vi "Acquire.Intermediary.vi"(7 "type":T1, 8 "error in":errorcluster, 10 "index":u64, 11 "camera.nit in":refnum<class "camera.lvclass">) -> (0 "error out":errorcluster, 2 "buffer":u16[][](array[numeric]))   [LabVIEW 2020, in "camera.lvclass"]
uses:
  camera.lvclass
  _controls/imageType.ctl
  camera.lvclass/camera.ctl
  lib/O-PL.dll
panel:
  out "Intensity Graph":u16[][](graph)
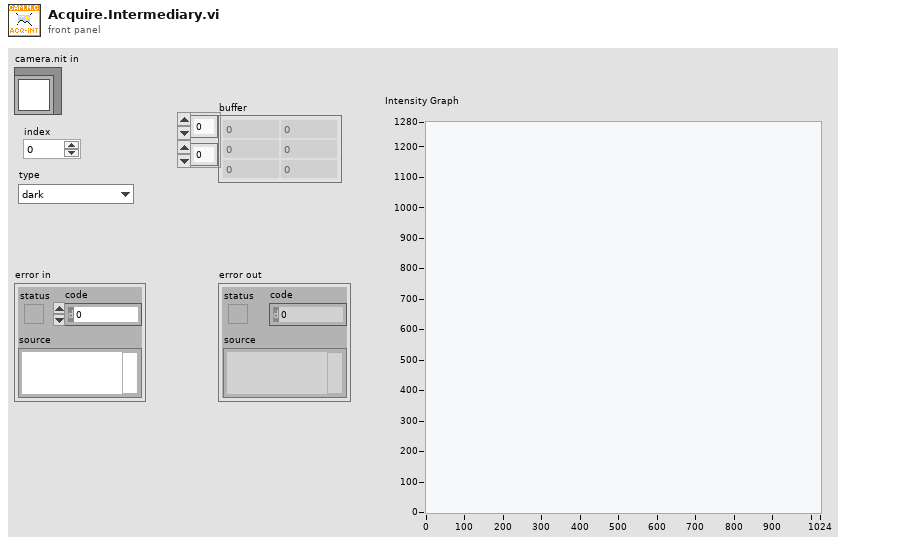
[diagram p1: front panel]
types:
  T1 = typedef "imageType.ctl" = enum16{"dark", "bright"}
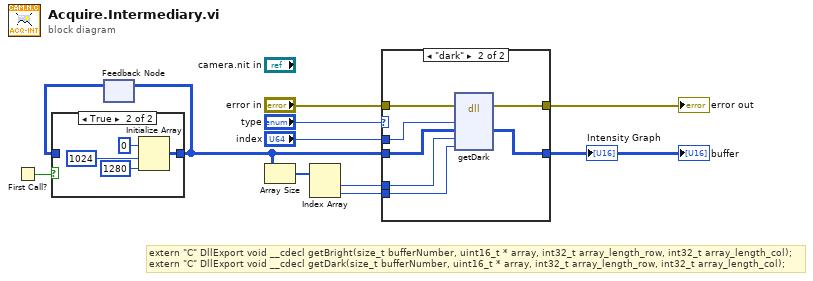
[diagram p0: block diagram]
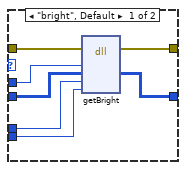
[diagram p2: hidden frame]
diagram:
  # "extern \"C\" DllExport void __cdecl getBright(size_t bufferNumber, uint16_t * array, int32_t array_length_row, int32_t array_length_col);\nextern \"C\" DllExport void __cdecl getDark(size_t bufferNumber, uint16_t * array, int32_t array_length_row, int32_t array_length_col);"
  n1 = First Call?() -> (First Call?: T/F=w9:bool)
  n2 = feedback #1() -> (w8:u16[][])  [unwired: 1 in]
  n3 = case shown="True" w9 {
    tunnel: w8 -> [w12 _]
    tunnel: [w12 w13] -> w5
    frame False {
    }
    frame True {
      n4 = Initialize Array(u16 0 ("element"), 1024 ("dimension size"), 1280 ("dimension size")) -> (w13:u16[][])
    }
  }
  n5 = feedback-in #1(w5) -> ()
  n6 = Array Size(array=w5) -> (size(s)=w7:i32[])
  n7 = Index Array(array=w7) -> (element #1=w4:i32, element #2=w6:i32)  [unwired: 2 in]
  n8 = case shown="\"dark\"" "type" {
    tunnel: w6 -> [w23 w30]
    tunnel: w5 -> [w22 w29]
    tunnel: w4 -> [w21 w28]
    tunnel: [w20 w27] -> w11
    tunnel: "error in" -> [w19 w26]
    tunnel: [w18 w25] -> w10
    tunnel: "index" -> [w17 w24]
    frame "bright", Default {
      n9 = dll-call lib="C:/Users/pittsburger.SOLARIS/Desktop/v0.8.1/lib/O-PL.dll" fn="getBright"(error in=w19, "bufferNumber"=w17, "array"=w22, "array_length_row"=w21, "array_length_col"=w23) -> (error out=w20:errorcluster, "array"=w18:u16[][])  [unwired: 4 in, 3 out]
    }
    frame "dark" {
      n10 = dll-call lib="C:/Users/pittsburger.SOLARIS/Desktop/v0.8.1/lib/O-PL.dll" fn="getDark"(error in=w26, "bufferNumber"=w24, "array"=w29, "array_length_row"=w28, "array_length_col"=w30) -> (error out=w27:errorcluster, "array"=w25:u16[][])  [unwired: 4 in, 3 out]
    }
  }
  "error out" <- w11
  "buffer" <- w10
  "Intensity Graph" <- w10
